vi "TrajectoryConfig_GetKinematicsSwerveDriveConstraint.vi"(11 "inTRAJECTORY_CONFIG":T1 {"End Velocity" format="%20.4f"; "StartVelocity" format="%20.4f"; "Max Acceleration" format="%20.4f"; "MaxVelocity" format="%20.4f"}) -> (1 "Constraint Exists":bool, 3 "Swerver Drive Kinematics Constraint":T2 {"SwerveKinematics"."PrevCoR"."Y" format="%14.3f"; "SwerveKinematics"."PrevCoR"."X" format="%14.3f"; "SwerveKinematics"."Modules"."Y" format="%14.3f"; "SwerveKinematics"."Modules"."X" format="%14.3f"; "Max Speed (M/S)" format="%20.4f"})   [LabVIEW 2019, in "Trajectory_Library.lvlib"]
doc: "Adds and enables a centripital acceleration constraint to ensure that the rotating capability of the robot is not exceeded.\n\nParameters:\n - MaxCentAccel - The maximum centripetal acceleration (meters/sec^2)\n - InTrajectoryConfig - The trajectory configuration data structure\n\nReturns:\n - OutTrajectoryConfig - Modified trajectory configuration data structure\n modified to conain them."
uses:
  Trajectory_Library.lvlib
  TypeDef/TRAJ_CONSTRAINT_SWERVE_DRIVE_KINEMATICS.ctl
  TypeDef/SWERVE_DRIVE_KINEMATICS.ctl
  <vilib>/Analysis/Matrix/Datatypes/RealMatrix.ctl
  TypeDef/TRANSLATION2D.ctl
  TypeDef/TRAJ_CONFIG.ctl
  <vilib>/Utility/Data Type/NI_Data Type.lvlib
  <vilib>/Analysis/Matrix/NI_Matrix.lvlib
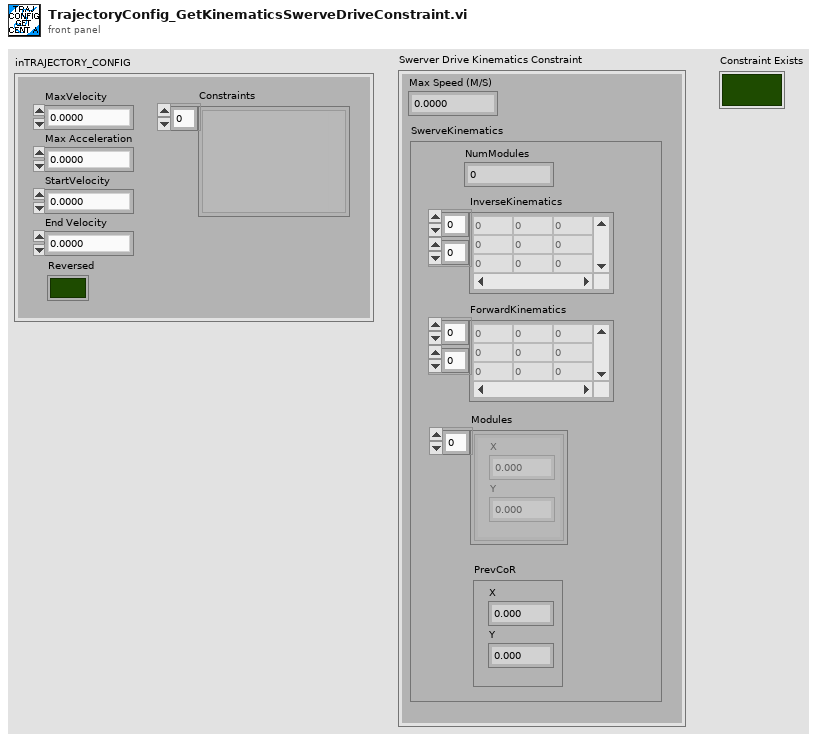
[diagram p1: front panel]
types:
  T1 = typedef "Trajectory_Library.lvlib/TRAJ_CONFIG.ctl" = cluster{"MaxVelocity":dbl, "Max Acceleration":dbl, "StartVelocity":dbl, "End Velocity":dbl, "Reversed":bool, "Constraints":variant[]}
  T2 = typedef "Trajectory_Library.lvlib/TRAJ_CONSTRAINT_SWERVE_DRIVE_KINEMATICS.ctl" = cluster{"Max Speed (M/S)":dbl, "SwerveKinematics":T3}
  T3 = typedef "Trajectory_Library.lvlib/SWERVE_DRIVE_KINEMATICS.ctl" = cluster{"NumModules":i32, "InverseKinematics":T4, "ForwardKinematics":T4, "Modules":T5[], "PrevCoR":T5}
  T4 = typedef "NI_Matrix.lvlib/RealMatrix.ctl" = dbl[][]
  T5 = typedef "Trajectory_Library.lvlib/TRANSLATION2D.ctl" = cluster{"X":dbl, "Y":dbl}
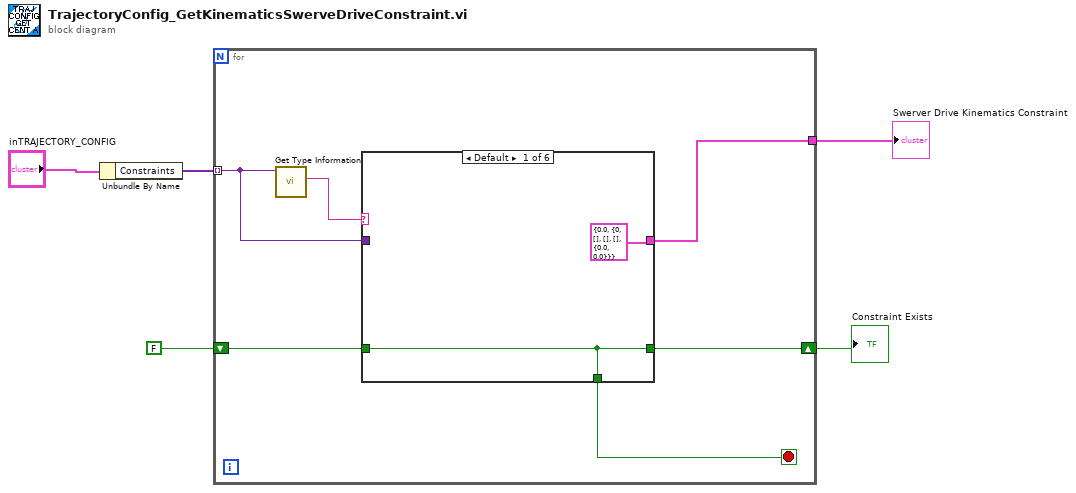
[diagram p0: block diagram]
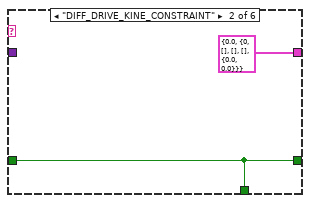
[diagram p2: hidden frame]
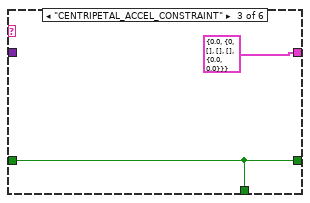
[diagram p3: hidden frame]
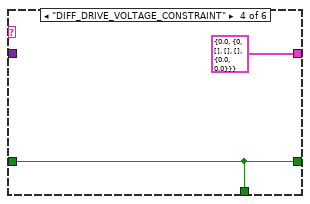
[diagram p4: hidden frame]
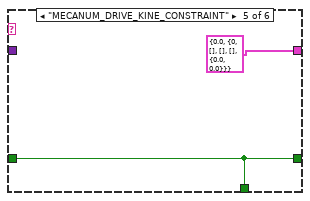
[diagram p5: hidden frame]
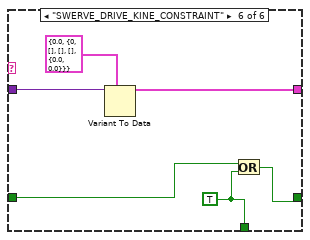
[diagram p6: hidden frame]
diagram:
  n1 = Unbundle By Name("inTRAJECTORY_CONFIG") -> ("Constraints"=w4:variant[])
  n2 = for {
    tunnel: w4 -> [w10] mode=indexing
    shift-right: [w8] -> w3
    shift-left: FALSE -> [w9]
    tunnel: [w7] -> w1
    stop <- w6 stop-if-true
    n3 = call <vilib>:"Get Type Information.vi"("variant"=w10) -> ("name"=w11:string)  [unwired: 6 in, 4 out]
    n4 = case shown="Default" w11 {
      tunnel: w10 -> [_ _ _ _ _ w26]
      tunnel: w9 -> [w12 w14 w16 w18 w20 w22]
      tunnel: [w12 w14 w16 w18 w20 w24] -> w8
      tunnel: [T2 {"Max Speed (M/S)"=0.0, "SwerveKinematics"={"NumModules"=0, "InverseKinematics"=[], "ForwardKinematics"=[], "Modules"=[], "PrevCoR"={"X"=0.0, "Y"=0.0}}} ("SWERVE_DRIVE_KINE_CONSTRAINT") T2 {"Max Speed (M/S)"=0.0, "SwerveKinematics"={"NumModules"=0, "InverseKinematics"=[], "ForwardKinematics"=[], "Modules"=[], "PrevCoR"={"X"=0.0, "Y"=0.0}}} ("SWERVE_DRIVE_KINE_CONSTRAINT") T2 {"Max Speed (M/S)"=0.0, "SwerveKinematics"={"NumModules"=0, "InverseKinematics"=[], "ForwardKinematics"=[], "Modules"=[], "PrevCoR"={"X"=0.0, "Y"=0.0}}} ("SWERVE_DRIVE_KINE_CONSTRAINT") T2 {"Max Speed (M/S)"=0.0, "SwerveKinematics"={"NumModules"=0, "InverseKinematics"=[], "ForwardKinematics"=[], "Modules"=[], "PrevCoR"={"X"=0.0, "Y"=0.0}}} ("SWERVE_DRIVE_KINE_CONSTRAINT") T2 {"Max Speed (M/S)"=0.0, "SwerveKinematics"={"NumModules"=0, "InverseKinematics"=[], "ForwardKinematics"=[], "Modules"=[], "PrevCoR"={"X"=0.0, "Y"=0.0}}} ("SWERVE_DRIVE_KINE_CONSTRAINT") w25] -> w7
      tunnel: [w12 w14 w16 w18 w20 w23] -> w6
      frame Default {
      }
      frame "DIFF_DRIVE_KINE_CONSTRAINT" {
      }
      frame "CENTRIPETAL_ACCEL_CONSTRAINT" {
      }
      frame "DIFF_DRIVE_VOLTAGE_CONSTRAINT" {
      }
      frame "MECANUM_DRIVE_KINE_CONSTRAINT" {
      }
      frame "SWERVE_DRIVE_KINE_CONSTRAINT" {
        w23 = TRUE
        n5 = Variant To Data(type=T2 {"Max Speed (M/S)"=0.0, "SwerveKinematics"={"NumModules"=0, "InverseKinematics"=[], "ForwardKinematics"=[], "Modules"=[], "PrevCoR"={"X"=0.0, "Y"=0.0}}} ("SWERVE_DRIVE_KINE_CONSTRAINT"), Variant=w26) -> (data=w25:T2)  [unwired: 1 in, 1 out]
        n6 = Or(x=w22, y=w23) -> (x .or. y?=w24:bool)
      }
    }
  }
  "Swerver Drive Kinematics Constraint" <- w1
  "Constraint Exists" <- w3
